vi "changeWavelengthDisplay.vi"(2 "X-Axis Unit":T1(ring)=enum."nanometer (nm)", 3 "Prev. Wavelength":dbl format="%.2f", 4 "Prev. Grating":enum16{"150", "300", "600", "1200", "1800"}(ring), 5 "New Grating Density":enum16{"150", "300", "600", "1200", "1800"}(ring)) -> (0 "New Wavelength output":dbl format="%.2f", 1 "Grating output":enum16{"150", "300", "600", "1200", "1800"}(ring)=enum."1200" caption="Current")   [LabVIEW 2021]
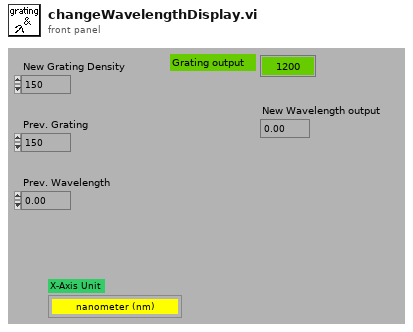
[diagram p1: front panel]
types:
  T1 = enum16{"Point #", "nanometer (nm)", "electron volt (eV)", "Milli eV (meV)", "Wavenumber (cm-1)"}
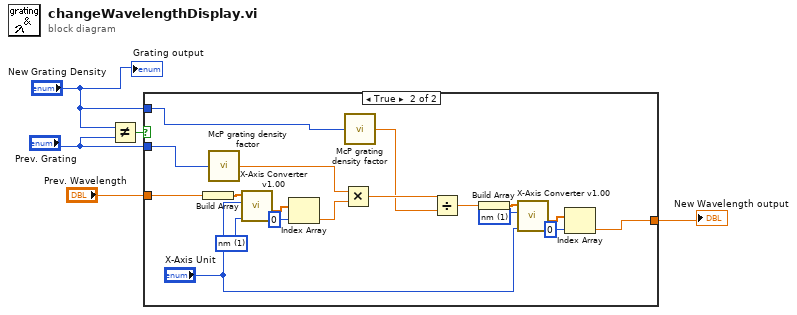
[diagram p0: block diagram]
diagram:
  n1 = Not Equal?(x="New Grating Density", y="Prev. Grating") -> (x != y?=w5:bool)
  n2 = case shown="True" w5 {
    tunnel: "Prev. Grating" -> [_ w11]
    tunnel: "New Grating Density" -> [_ w8]
    tunnel: "Prev. Wavelength" -> [w6 w13]
    tunnel: [w6 w12] -> w1
    frame False {
    }
    frame True {
      w14 = 1 items=["Point #", "nm", "eV", "meV", "cm-1"] ("Old X-Axis Unit")
      w22 = 1 items=["Point #", "nm", "eV", "meV", "cm-1"] ("X-Axis Unit")
      n3 = Build Array(w13) -> (w24:dbl[])
      n4 = call "McP grating density factor.vi"("Grating Density"=w11) -> ("GratingFactor"=w10:dbl)
      n5 = call "X-Axis Converter v1.00.vi"("X-Axis Unit"=w22, "Old X-Axis Unit"="X-Axis Unit", "X-Axis input"=w24) -> ("X-Axis Output"=w23:dbl[])  [unwired: 2 in, 3 out]
      n6 = Index Array(array=w23, index=0) -> (element=w21:dbl)
      n7 = Multiply(x=w10, y=w21) -> (x*y=w19:dbl)
      n8 = call "McP grating density factor.vi"("Grating Density"=w8) -> ("GratingFactor"=w9:dbl)
      n9 = Divide(x=w19, y=w9) -> (x/y=w18:dbl)
      n10 = Build Array(w18) -> (w17:dbl[])
      n11 = call "X-Axis Converter v1.00.vi"("X-Axis Unit"="X-Axis Unit", "Old X-Axis Unit"=w14, "X-Axis input"=w17) -> ("X-Axis Output"=w16:dbl[])  [unwired: 2 in, 3 out]
      n12 = Index Array(array=w16, index=0) -> (element=w12:dbl)
    }
  }
  "New Wavelength output" <- w1
  "Grating output" <- "New Grating Density"
